vi "Write Vss Skills.vi"(8 "error in (no error)":errorcluster, 10 "Vss Skills":T1, 11 "Skillbook in":refnum<class "Skillbook.lvclass">) -> (0 "error out":errorcluster, 3 "Skillbook out":refnum<class "Skillbook.lvclass">)   [LabVIEW 2023, in "Skillbook.lvclass"]
uses:
  Skillbook.lvclass
  KickSkillVSS_class/KickSkillVSS.lvclass
  PenaltyPosSkillVSS_class/PenaltyPosSkillVSS.lvclass
  BallDispPosSkillVSS_class/BallDispPosSkillVSS.lvclass
  BallToGoalSkillVSS_class/BallToGoalSkillVSS.lvclass
  GoToBallSkillVSS_class/GoToBallSkillVSS.lvclass
  DefBallPosSkillVSS_class/DefBallPosSkillVSS.lvclass
  HaltSkill_class/HaltSkill.lvclass
  KeeperDefPosSkillVSS_class/KeeperDefPosSkillVSS.lvclass
  GoToBallKeeperSkillVSS_class/GoToBallKeeperSkillVSS.lvclass
  RotateWallSkillVSS_class/RotateWallSkillVSS.lvclass
  Skillbook.lvclass/Skillbook.ctl
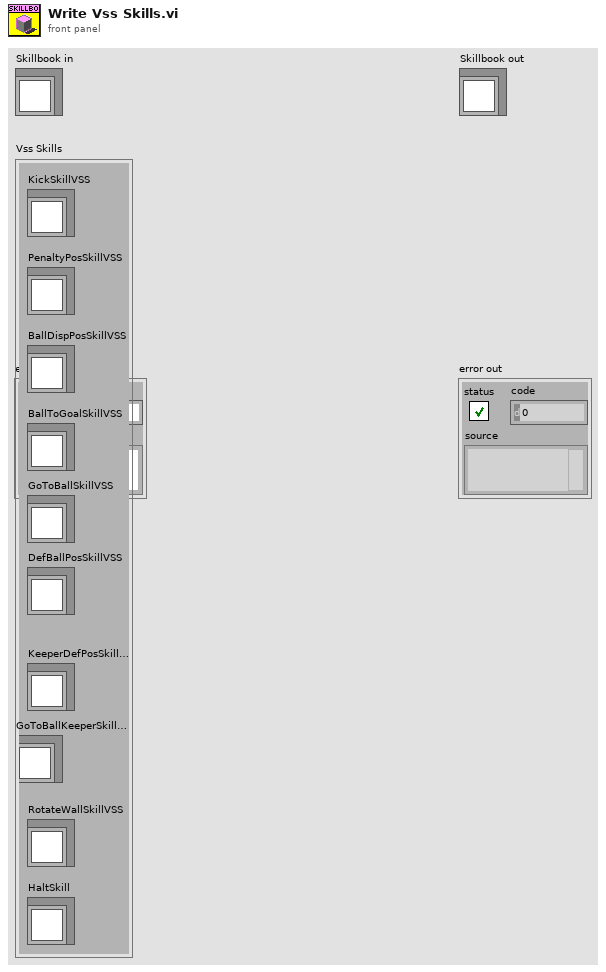
[diagram p1: front panel]
types:
  T1 = cluster{"KickSkillVSS":refnum<class "KickSkillVSS.lvclass">, "PenaltyPosSkillVSS":refnum<class "PenaltyPosSkillVSS.lvclass">, "BallDispPosSkillVSS":refnum<class "BallDispPosSkillVSS.lvclass">, "BallToGoalSkillVSS":refnum<class "BallToGoalSkillVSS.lvclass">, "GoToBallSkillVSS":refnum<class "GoToBallSkillVSS.lvclass">, "DefBallPosSkillVSS":refnum<class "DefBallPosSkillVSS.lvclass">, "HaltSkill":refnum<class "HaltSkill.lvclass">, "KeeperDefPosSkillVSS":refnum<class "KeeperDefPosSkillVSS.lvclass">, "GoToBallKeeperSkillVSS":refnum<class "GoToBallKeeperSkillVSS.lvclass">, "RotateWallSkillVSS":refnum<class "RotateWallSkillVSS.lvclass">}
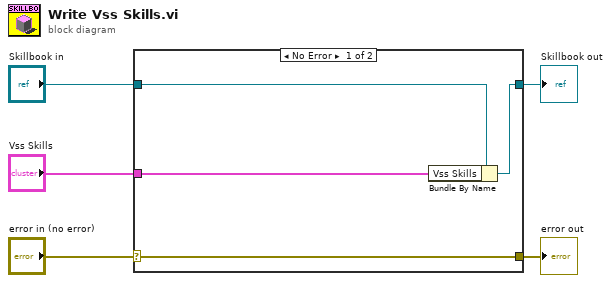
[diagram p0: block diagram]
diagram:
  n1 = case shown="No Error" "error in (no error)" {
    selector: "error in (no error)" -> [w9 w10]
    tunnel: [w9 w10] -> w4
    tunnel: [w7 w11] -> w2
    tunnel: "Skillbook in" -> [w8 w11]
    tunnel: "Vss Skills" -> [w6 _]
    frame No Error {
      n2 = Bundle By Name(cluster=w8, "Vss Skills"=w6) -> (w7:refnum<class "Skillbook.lvclass">)
    }
    frame Error {
    }
  }
  "error out" <- w4
  "Skillbook out" <- w2
